vi "AND.vi"() -> ()   [LabVIEW 2021]
panel:
  out "A1 and B1":u8 format="%b"
  in  "B1":u8 format="%b"
  in  "A1":u8 format="%b"
  out "A .and. B":bool
  in  "B":bool
  in  "A":bool
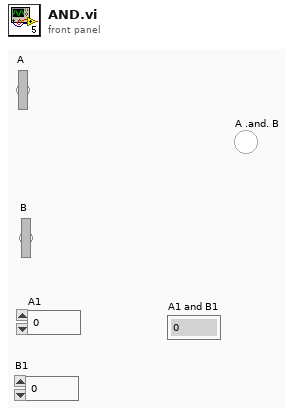
[diagram p1: front panel]
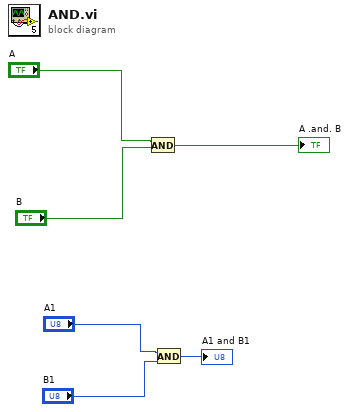
[diagram p0: block diagram]
diagram:
  n1 = And(x="A", y="B") -> (x .and. y?=→"A .and. B":bool)
  n2 = And(x="A1", y="B1") -> (x .and. y?=→"A1 and B1":u8)
